vi "Lower Cascade Requested.vi"(7 "Delay?":bool, 10 "Score Requested?":bool, 11 "Reset?":bool) -> (3 "Lower Cascade?":bool)   [LabVIEW 2020]
uses:
  88aedc65-fd34-4979-806e-4511f7ca64b4.vi
  f02d2be1-34e2-401b-a77e-a40bef360958.vi
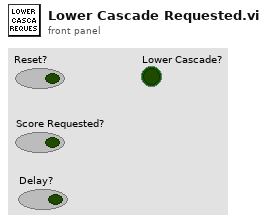
[diagram p1: front panel]
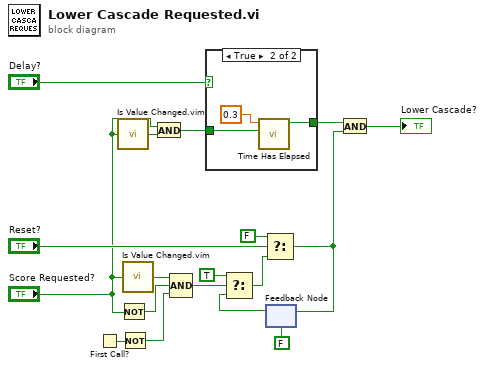
[diagram p0: block diagram]
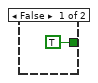
[diagram p2: hidden frame]
diagram:
  n1 = First Call?() -> (First Call?: T/F=w9:bool)
  n2 = call "Is Value Changed.vim"("value"="Score Requested?") -> ("changed or first call?"=w6:bool)
  n3 = Not(x="Score Requested?") -> (.not. x?=w11:bool)
  n4 = Not(x=w9) -> (.not. x?=w8:bool)
  n5 = call "Is Value Changed.vim"("value"="Score Requested?") -> ("changed or first call?"=w12:bool)
  n6 = And(x="Score Requested?", y=w6) -> (x .and. y?=w4:bool)
  n7 = Compound Arithmetic op=AND(w12, w11, w8) -> (w10:bool)
  n8 = case shown="True" "Delay?" {
    tunnel: w4 -> [_ w22]
    tunnel: [TRUE ("Elapsed Time Passed?") w21] -> w1
    frame False {
    }
    frame True {
      n9 = call "Time Has Elapsed.vi"("Reset?"=w22, "Delay"=0.3) -> ("Elapsed Time Passed?"=w21:bool)  [unwired: 8 in, 1 out]
    }
  }
  n10 = feedback #1(FALSE) -> (w17:bool)
  n11 = Select(t=TRUE, s=w10, f=w17) -> (s? t:f=w13:bool)
  n12 = Select(t=FALSE, s="Reset?", f=w13) -> (s? t:f=w2:bool)
  n13 = feedback-in #1(w2) -> ()
  n14 = And(x=w1, y=w2) -> (x .and. y?=→"Lower Cascade?":bool)
